vi "FCE_TS_Action_InitGlobals.vi"(8 "err in":errorcluster) -> (0 "err out":errorcluster)   [LabVIEW 2017]
uses:
  FCE_TS_State_V001.llb/FCE_TS_State_TDefEnumGlobalState.ctl
  FCE_TS_State_V001.llb/FCE_TS_State_TDefEnumStateDatalog.ctl
  FCE_TS_General_Libs/WL_Libs_V14.25/WL_Frontpanel_V14.01.llb/WL_Frontpanel_GblStatus.vi
  FCE_TS_Globals_V001.llb/FCE_TS_Globals_Status.vi
  FCE_TS_Globals_V001.llb/FCE_TS_Globals_Action.vi
  FCE_TS_State_V001.llb/FCE_TS_State_Globals.vi
  FCE_TS_General_Libs/WL_Libs_V14.25/WL_Profile_V14.00.llb/WL_Profile_Globals.vi
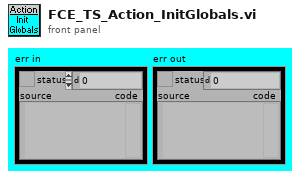
[diagram p1: front panel]
types:
  T1 = typedef "FCE_TS_State_TDefEnumStateDatalog.ctl" = enum16{"default", "StartLog", "Log", "StopLog", "NewFile"}
  T2 = typedef "FCE_TS_State_TDefEnumGlobalState.ctl" = enum16{"System_Off", "Initialize", "Standby", "H2-On", "Shutdown", "Alarm", "Component_Test"}
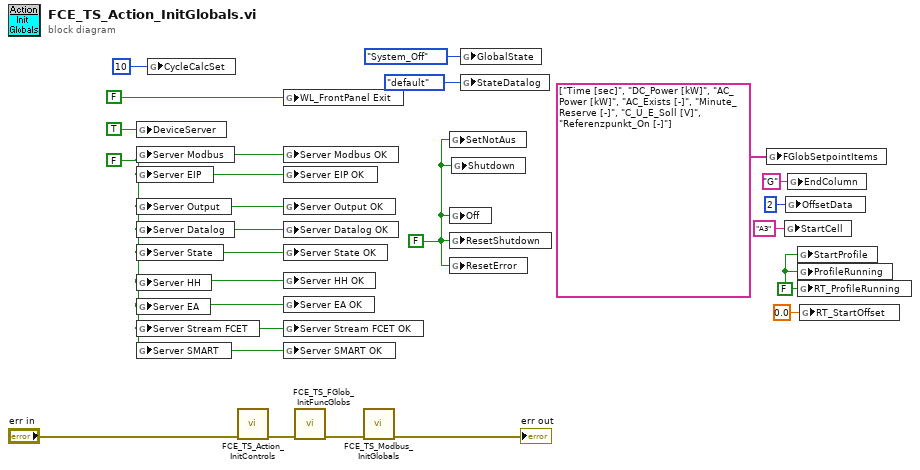
[diagram p0: block diagram]
diagram:
  w5 = FALSE ("RT_ProfileRunning")
  w10 = FALSE ("Purge_Man")
  w1 = FALSE ("Server Alarm")
  n1 = global write "FCE_TS_Globals_Status.vi" "DeviceServer"(TRUE ("DeviceServer")) -> ()
  n2 = global write "FCE_TS_Globals_Action.vi" "Server Modbus"(w1) -> ()
  n3 = global write "FCE_TS_Globals_Action.vi" "Server EIP"(w1) -> ()
  n4 = global write "FCE_TS_Globals_Action.vi" "Server Output"(w1) -> ()
  n5 = global write "FCE_TS_Globals_Action.vi" "Server Datalog"(w1) -> ()
  n6 = global write "FCE_TS_Globals_Action.vi" "Server State"(w1) -> ()
  n7 = global write "FCE_TS_Globals_Action.vi" "Server HH"(w1) -> ()
  n8 = global write "FCE_TS_Globals_Action.vi" "Server EA"(w1) -> ()
  n9 = global write "FCE_TS_Globals_Action.vi" "Server Stream FCET"(w1) -> ()
  n10 = global write "FCE_TS_Globals_Action.vi" "Server SMART"(w1) -> ()
  n11 = global write "FCE_TS_Globals_Action.vi" "CycleCalcSet"(u32 10 ("CycleCalcSet")) -> ()
  n12 = call "FCE_TS_Action_InitControls.vi"("err in"="err in") -> ("err out"=w15:errorcluster)  [unwired: 10 in]
  n13 = global write "WL_Frontpanel_GblStatus.vi" "WL_FrontPanel Exit"(FALSE ("BL_FrontPanel Exit")) -> ()
  n14 = global write "FCE_TS_Globals_Action.vi" "Server Modbus OK"(w1) -> ()
  n15 = global write "FCE_TS_Globals_Action.vi" "Server EIP OK"(w1) -> ()
  n16 = global write "FCE_TS_Globals_Action.vi" "Server Output OK"(w1) -> ()
  n17 = global write "FCE_TS_Globals_Action.vi" "Server Datalog OK"(w1) -> ()
  n18 = global write "FCE_TS_Globals_Action.vi" "Server State OK"(w1) -> ()
  n19 = global write "FCE_TS_Globals_Action.vi" "Server HH OK"(w1) -> ()
  n20 = global write "FCE_TS_Globals_Action.vi" "Server EA OK"(w1) -> ()
  n21 = global write "FCE_TS_Globals_Action.vi" "Server Stream FCET OK"(w1) -> ()
  n22 = global write "FCE_TS_Globals_Action.vi" "Server SMART OK"(w1) -> ()
  n23 = call "FCE_TS_FGlob_InitFuncGlobs.vi"("err in"=w15) -> ("err out"=w3:errorcluster)  [unwired: 10 in]
  n24 = call "FCE_TS_Modbus_InitGlobals.vi"("err in"=w3) -> ("err out"=→"err out":errorcluster)  [unwired: 10 in]
  n25 = global write "FCE_TS_Globals_Action.vi" "SetNotAus"(w10) -> ()
  n26 = global write "FCE_TS_Globals_Action.vi" "Off"(w10) -> ()
  n27 = global write "FCE_TS_Globals_Action.vi" "ResetShutdown"(w10) -> ()
  n28 = global write "FCE_TS_Globals_Action.vi" "ResetError"(w10) -> ()
  n29 = global write "FCE_TS_Globals_Action.vi" "Shutdown"(w10) -> ()
  n30 = global write "FCE_TS_State_Globals.vi" "GlobalState"(FCE_TS_State_TDefEnumGlobalState."System_Off" ("GlobalState")) -> ()
  n31 = global write "FCE_TS_State_Globals.vi" "StateDatalog"(FCE_TS_State_TDefEnumStateDatalog."default" ("StateDatalog")) -> ()
  n32 = global write "WL_Profile_Globals.vi" "FGlobSetpointItems"(string[] ["Time [sec]", "DC_Power [kW]", "AC_Power [kW]", "AC_Exists [-]", "Minute_Reserve [-]", "C_U_E_Soll [V]", "Referenzpunkt_On [-]"] ("FGlobSetpointItems")) -> ()
  n33 = global write "WL_Profile_Globals.vi" "StartCell"("A3" ("StartCell")) -> ()
  n34 = global write "WL_Profile_Globals.vi" "OffsetData"(2 ("OffsetData")) -> ()
  n35 = global write "WL_Profile_Globals.vi" "EndColumn"("G" ("EndColumn")) -> ()
  n36 = global write "WL_Profile_Globals.vi" "StartProfile"(w5) -> ()
  n37 = global write "WL_Profile_Globals.vi" "ProfileRunning"(w5) -> ()
  n38 = global write "WL_Profile_Globals.vi" "RT_ProfileRunning"(w5) -> ()
  n39 = global write "WL_Profile_Globals.vi" "RT_StartOffset"(sgl 0.0 ("RT_StartOffset")) -> ()
